vi "Get User Interface Information.vi"(8 "error in (no error)":errorcluster, 11 "measurement plugin in":refnum<class "Signal Simulator Plug-In.lvclass">) -> (0 "error out":errorcluster, 2 "user interface information":cluster{"file":string}[](array[cluster]), 3 "measurement plugin out":refnum<class "Signal Simulator Plug-In.lvclass">)   [LabVIEW 2026, in "Signal Simulator Plug-In.lvclass"]
doc: "Returns the UI files InstrumentStudio shows: the Measurement Plug-In UI (.measui) first, then the LabVIEW front panel as an alternative."
uses:
  Signal Simulator Plug-In.lvclass
  Signal Simulator Plug-In.lvclass/Signal Simulator Plug-In.ctl
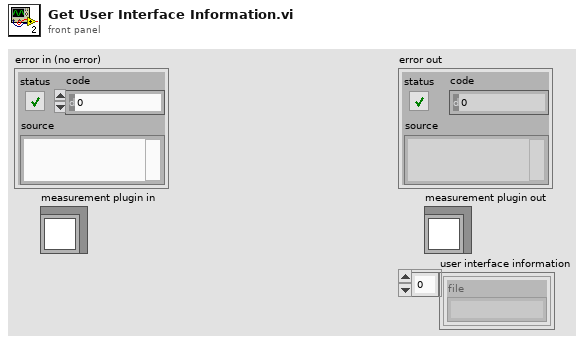
[diagram p1: front panel]
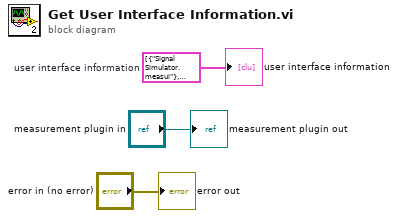
[diagram p0: block diagram]
diagram:
  w1 = cluster{"file":string}[] [{"file"="Signal Simulator.measui"}, {"file"="BuiltUI\\Signal Simulator Plug-In UI.lvlibp\\Measurement UI.vi"}]  # user interface information
  "error out" <- "error in (no error)"
  "measurement plugin out" <- "measurement plugin in"
  "user interface information" <- w1
